vi "getAndorErrorCodes.vi"(8 "error in (no error)":errorcluster, 11 "AndorIKonTempController.lvclass in":refnum<class "AndorIKonTempController.lvclass">) -> (0 "error out":errorcluster, 2 "Andor Error Codes":dbl[](array[numeric]), 3 "AndorIKonTempController.lvclass out":refnum<class "AndorIKonTempController.lvclass">)   [LabVIEW 2011, in "Hardware.lvlib" / "Channels.lvlib" / "AndorIKonTempController.lvclass"]
uses:
  AndorIKonTempController.lvclass
  AndorIKonTempController.lvclass/AndorIKonTempController.ctl
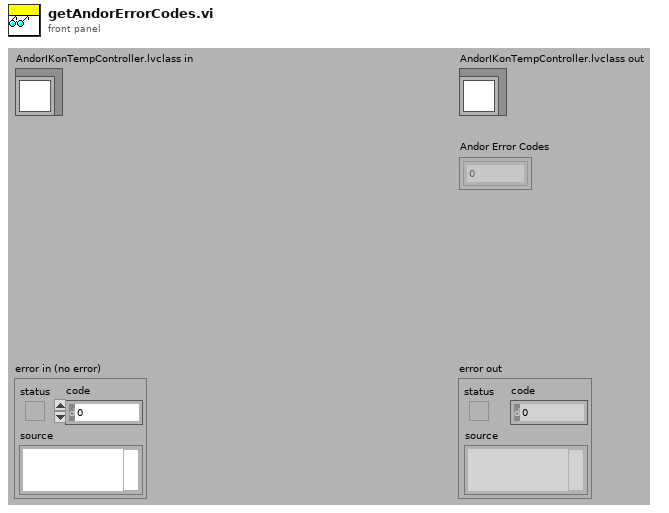
[diagram p1: front panel]
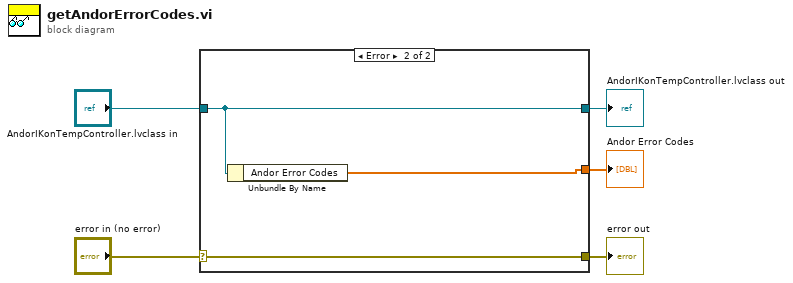
[diagram p0: block diagram]
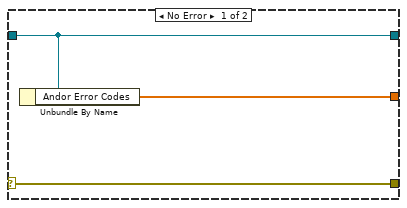
[diagram p2: hidden frame]
diagram:
  n1 = case shown="Error" "error in (no error)" {
    selector: "error in (no error)" -> [w8 w11]
    tunnel: [w8 w11] -> w4
    tunnel: [w7 w10] -> w2
    tunnel: "AndorIKonTempController.lvclass in" -> [w7 w10]
    tunnel: [w6 w9] -> w1
    frame No Error {
      n2 = Unbundle By Name(w7) -> ("Andor Error Codes"=w6:dbl[])
    }
    frame Error {
      n3 = Unbundle By Name(w10) -> ("Andor Error Codes"=w9:dbl[])
    }
  }
  "error out" <- w4
  "AndorIKonTempController.lvclass out" <- w2
  "Andor Error Codes" <- w1
